vi "Obtain ByRef (Unnamed SEQ).vi"(8 "error in (no error)":errorcluster, 11 "Numeric in":refnum<class "Numeric Test Object.lvclass">) -> (0 "error out":errorcluster, 3 "Numeric out":refnum<class "Numeric Test Object.lvclass">)   [LabVIEW 2009, in "Numeric Test Object.lvclass"]
doc: "Obtains a reference to a SEQ and stores it in the class cluster."
uses:
  Numeric Test Object.lvclass
  Numeric Test Object.lvclass/Numeric Test Object.ctl
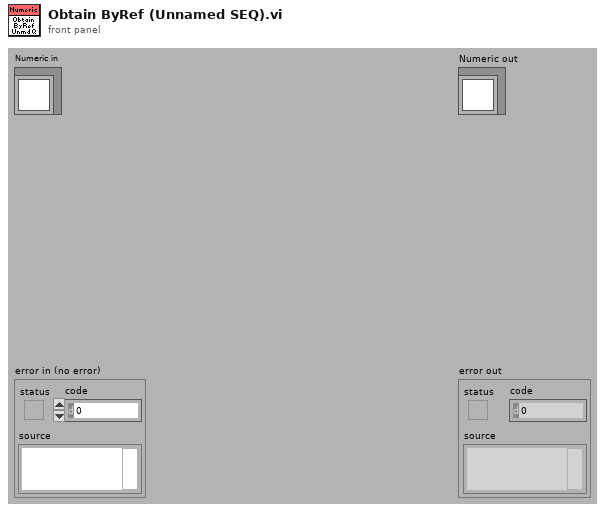
[diagram p1: front panel]
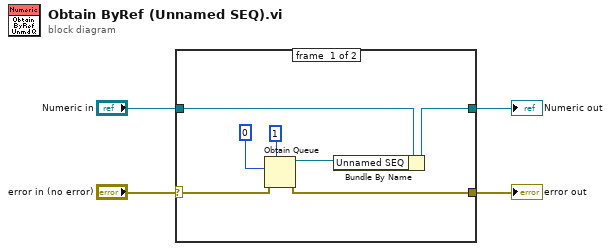
[diagram p0: block diagram]
diagram:
  n1 = case shown="No Error" "error in (no error)" {
    selector: "error in (no error)" -> [w10 w13]
    tunnel: [w5 w13] -> w3
    tunnel: [w11 w12] -> w1
    tunnel: "Numeric in" -> [w7 w12]
    frame #0 {
      n2 = Obtain Queue(max queue size (-1, unlimited)=1, element data type=0, error in (no error)=w10) -> (queue out=w6:refnum<queue>, error out=w5:errorcluster)  [unwired: 2 in, 1 out]
      n3 = Bundle By Name(cluster=w7, "Unnamed SEQ"=w6) -> (w11:refnum<class "Numeric Test Object.lvclass">)
    }
    frame #1 {
    }
  }
  "error out" <- w3
  "Numeric out" <- w1
